vi "myRIO_BRig_RT_dataExp_laser2_Tpeak.vi"() -> (2 "output_laser2_Tpeak":i32)   [LabVIEW 2014]
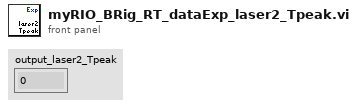
[diagram p1: front panel]
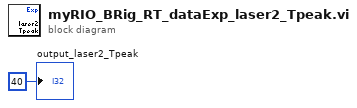
[diagram p0: block diagram]
diagram:
  "output_laser2_Tpeak" <- 40 ("output_iBlock")
